vi "getSettingsEventsManager.vi"(8 "error in (no error)":errorcluster, 11 "CameraEventsManger.lvclass in":refnum<class "CameraEventsManger.lvclass">) -> (0 "error out":errorcluster, 2 "SettingsEventsManager":refnum<class "SettingsEventsManager.lvclass">, 3 "CameraEventsManger.lvclass out":refnum<class "CameraEventsManger.lvclass">)   [LabVIEW 2011, in "Tools.lvlib" / "Settings.lvlib" / "CameraEventsManger.lvclass"]
uses:
  CameraEventsManger.lvclass
  Tools/SettingsEventManager/SettingsEventsManager.lvclass
  CameraEventsManger.lvclass/CameraEventsManger.ctl
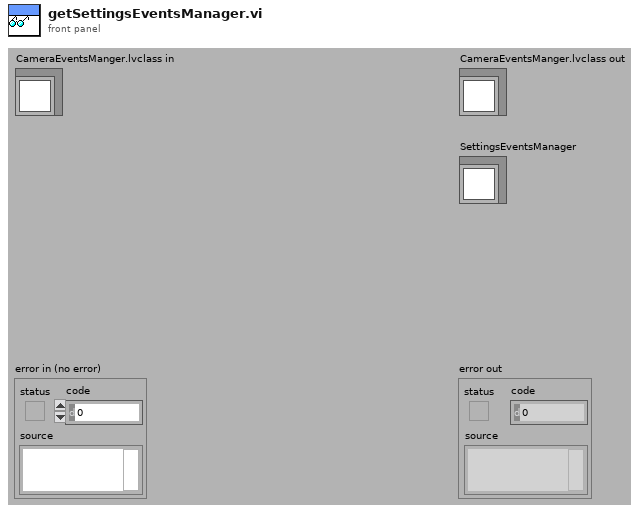
[diagram p1: front panel]
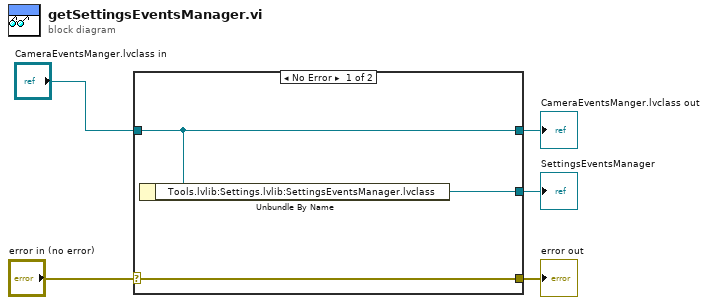
[diagram p0: block diagram]
diagram:
  n1 = case shown="No Error" "error in (no error)" {
    selector: "error in (no error)" -> [w8 w9]
    tunnel: [w8 w9] -> w4
    tunnel: [w7 w10] -> w2
    tunnel: "CameraEventsManger.lvclass in" -> [w7 w10]
    tunnel: [w6 _] -> w1
    frame No Error {
      n2 = Unbundle By Name(w7) -> ("Tools.lvlib:Settings.lvlib:SettingsEventsManager.lvclass"=w6:refnum<class "SettingsEventsManager.lvclass">)
    }
    frame Error {
    }
  }
  "error out" <- w4
  "CameraEventsManger.lvclass out" <- w2
  "SettingsEventsManager" <- w1
